vi "Stop Core.vi"(10 "final error code":i32, 11 "CS++DeviceGUIActor in":refnum<class "CS++DIM-Client.lvclass">) -> (3 "CS++DeviceGUIActor out":refnum<class "CS++DIM-Client.lvclass">)   [LabVIEW 2014, in "CS++DIM-Client.lvlib" / "CS++DIM-Client.lvclass"]
doc: "(<B>Filename</B>: Actor Framework.lvlib:Actor.lvclass:Stop Core.vi)\n\nDefines what the actor does before it stops. Use the <B>final error code</B> input to determine whether the actor shut down in response to an error.\n\nBy default, this method does nothing. A descendant class may override it to define behavior, such as shutting down any processes the actor initiated in its override of the Actor Core method."
uses:
  CS++DIM-Client.lvclass
  CS++DIM-Client.lvclass/CS++DIM-Client.ctl
  CSPP_Core/Actors/CS++GUIActor/CS++GUIActor.lvclass
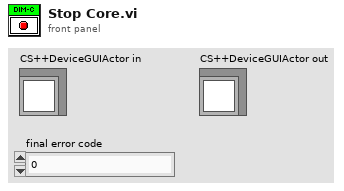
[diagram p1: front panel]
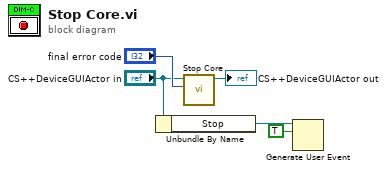
[diagram p0: block diagram]
diagram:
  n1 = Unbundle By Name("CS++DeviceGUIActor in") -> ("Stop"=w1:refnum<user-event>)
  n2 = call-parent "Stop Core.vi"("final error code"="final error code", "CS++DeviceGUIActor in"="CS++DeviceGUIActor in") -> ("CS++DeviceGUIActor out"=→"CS++DeviceGUIActor out":refnum<class "CS++DIM-Client.lvclass">)  [unwired: 9 in]
  n3 = Generate User Event(user event=w1, event data cluster=TRUE ("event data")) -> ()  [unwired: 2 in, 2 out]
